vi "GFITS_getKeyvalueFromDatabase.vi"(0 "key name in header":string, 1 "Database RefNum in":T1, 5 "Keyname":string, 7 "comment":string, 9 "extension":i16=1, 11 "error in (no error)":errorcluster) -> (6 "table out":string[][](table), 10 "datatype":u16[](array[numeric]), 14 "function to use":string, 15 "error out":errorcluster)   [LabVIEW 2016]
uses:
  GFITS_datatypesctl.ctl
  DBSHAND/private/vis/DatabaseHand_RefNum.ctl
  DBSHAND/private/vis/DatabaseHand_Element_Get(string).vi
  GFITS_Gbls.vi
  DBSHAND/private/vis/DatabaseHand_Element_Get(3DArr).vi
panel:
  in  "Case Constant\n(See Context Help)":bool
  out "TCSINFO":string[][](array[string])
  in  "ARRINFO":string[][](table)
  out "value":string
  out "response":string
  out "utshut":string
  in  "Types":T2={"TBIT"=1, "TBYTE"=11, "TSTRING"=16, "TSHORT"=21, "TLONG"=41, "TFLOAT"=42, "TDOUBLE"=82, "TCOMPLEX"=83, "TDBLCOMPLEX"=163, "TUINT"=30, "TUSHORT"=20, "TULONG"=40, "TINT"=31, "TSBYTE"=12, "TLONGLONG"=81, "TLOGICAL"=14}
  in  "Supported DataTypes":i32(listbox)
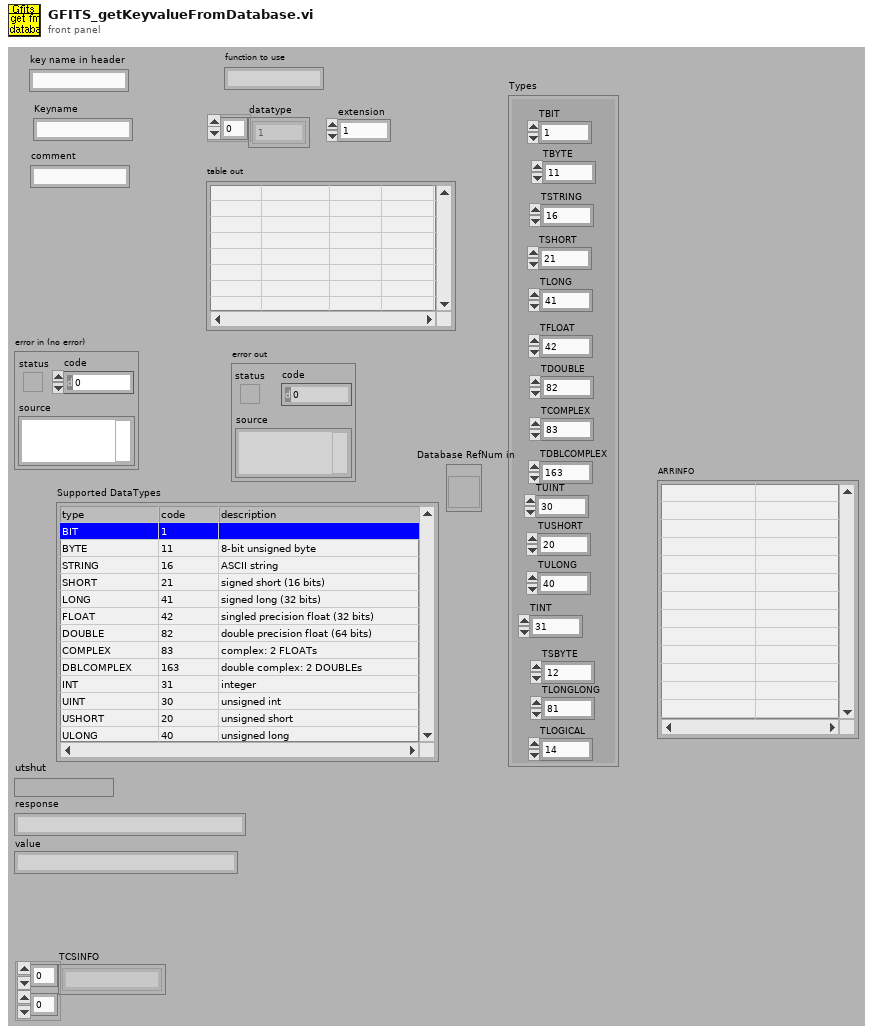
[diagram p1: front panel]
types:
  T1 = typedef "DatabaseHand_RefNum.ctl" = refnum<vi>
  T2 = typedef "GFITS_datatypesctl.ctl" = cluster{"TBIT":i32, "TBYTE":i32, "TSTRING":i32, "TSHORT":i32, "TLONG":i32, "TFLOAT":i32, "TDOUBLE":i32, "TCOMPLEX":i32, "TDBLCOMPLEX":i32, "TUINT":i32, "TUSHORT":i32, "TULONG":i32, "TINT":i32, "TSBYTE":i32, "TLONGLONG":i32, "TLOGICAL":i32}
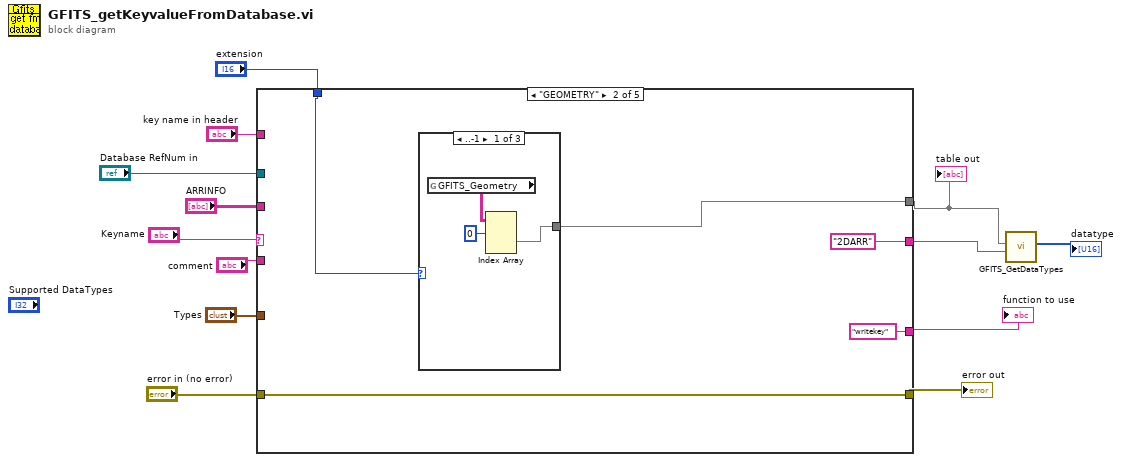
[diagram p0: block diagram]
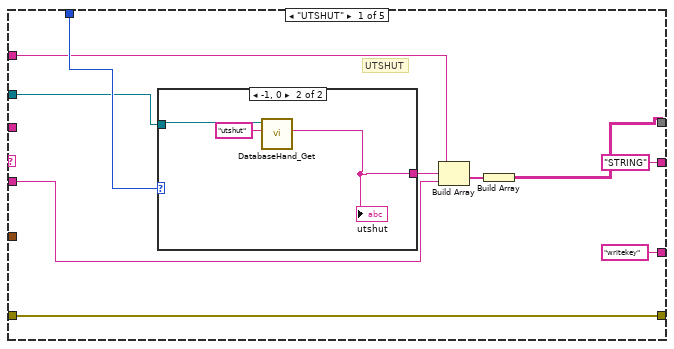
[diagram p2: hidden frame]
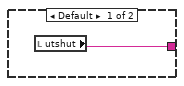
[diagram p3: hidden frame]
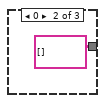
[diagram p4: hidden frame]
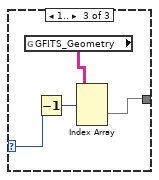
[diagram p5: hidden frame]
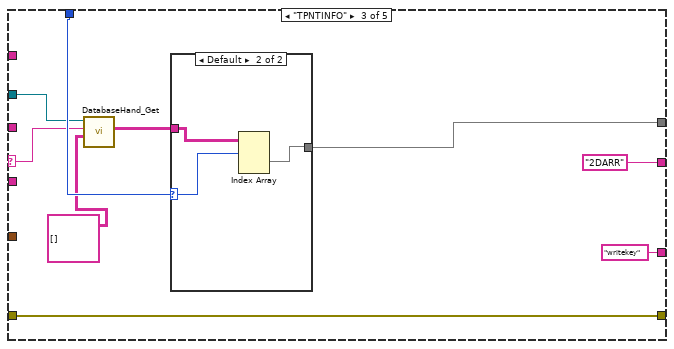
[diagram p6: hidden frame]
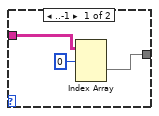
[diagram p7: hidden frame]
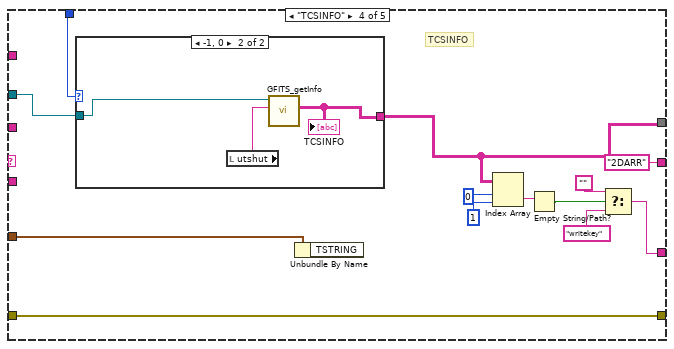
[diagram p8: hidden frame]
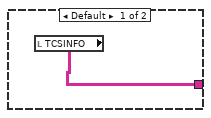
[diagram p9: hidden frame]
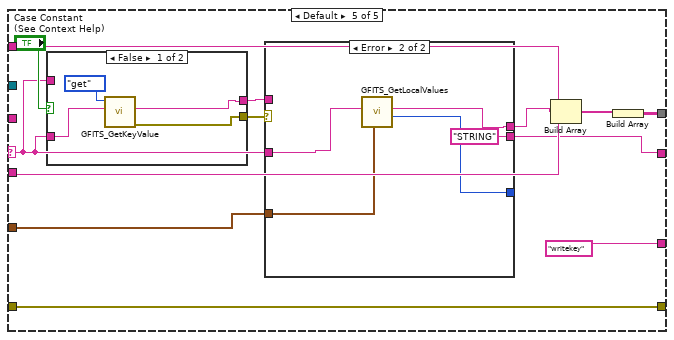
[diagram p10: hidden frame]
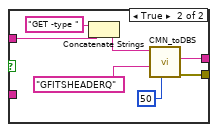
[diagram p11: hidden frame]
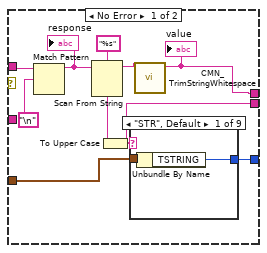
[diagram p12: hidden frame]
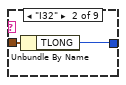
[diagram p13: hidden frame]
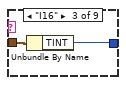
[diagram p14: hidden frame]
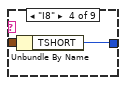
[diagram p15: hidden frame]
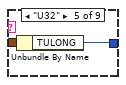
[diagram p16: hidden frame]
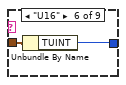
[diagram p17: hidden frame]
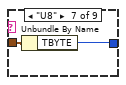
[diagram p18: hidden frame]
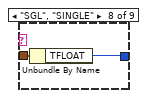
[diagram p19: hidden frame]
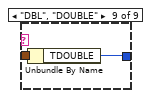
[diagram p20: hidden frame]
diagram:
  n1 = case shown="\"GEOMETRY\"" "Keyname" {
    selector: "Keyname" -> [_ _ w43 _ w74]
    tunnel: "key name in header" -> [w20 _ _ _ w83]
    tunnel: "comment" -> [w19 _ _ _ w82]
    tunnel: "error in (no error)" -> [w17 w32 w49 w68 w85]
    tunnel: [w17 w32 w49 w68 w85] -> w10
    tunnel: ["writekey" "writekey" "writekey" w65 "writekey"] -> w9
    tunnel: [w18 w29 w46 w60 w81] -> w2
    tunnel: "extension" -> [w21 w30 w47 w64 _]
    tunnel: "Types" -> [_ _ _ w58 w78]
    tunnel: "ARRINFO" -> [_ _ _ _ _]
    tunnel: "Database RefNum in" -> [w15 _ w44 w56 _]
    tunnel: ["STRING" ("type") "2DARR" ("type") "2DARR" ("type") "2DARR" ("type") w73] -> w1
    frame "UTSHUT" {
      # "UTSHUT"
      n2 = case shown="-1, 0" w21 {
        tunnel: [w24 w25] -> w22
        tunnel: w15 -> [_ w27]
        frame Default {
          n3 = local read "utshut"() -> (w24:string)
        }
        frame -1, 0 {
          n4 = call-poly "DatabaseHand_Get.vi"("name"="utshut", "Database RefNum in"=w27) -> ("value"=w25:string)  [unwired: 3 in, 6 out]
          "utshut" <- w25
        }
      }
      n5 = Build Array(w20, w22, w19) -> (w23:string[])
      n6 = Build Array(w23) -> (w18:string[][])
    }
    frame "GEOMETRY" {
      n7 = case shown="..-1" w30 {
        selector: w30 -> [_ _ w39]
        tunnel: [w33 string[][] [] ("GFITS_Geometry") w38] -> w29
        frame ..-1 {
          n8 = global read "GFITS_Gbls.vi" "GFITS_Geometry"() -> (w35:string[][][])
          n9 = Index Array(array=w35, index (dim 0)=0 ("index (page)")) -> (element=w33:string[][])  [unwired: 2 in]
        }
        frame 0 {
        }
        frame 1.. {
          n10 = global read "GFITS_Gbls.vi" "GFITS_Geometry"() -> (w40:string[][][])
          n11 = Decrement(x=w39) -> (x-1=w37:i16)
          n12 = Index Array(array=w40, index (dim 0)=w37) -> (element=w38:string[][])  [unwired: 2 in]
        }
      }
    }
    frame "TPNTINFO" {
      n13 = call-poly "DatabaseHand_Get.vi"("default value"=string[][][] [] ("GFITS_Geometry"), "name"=w43, "Database RefNum in"=w44) -> ("value"=w41:string[][][])  [unwired: 2 in, 6 out]
      n14 = case shown="Default" w47 {
        selector: w47 -> [_ w54]
        tunnel: [w51 w55] -> w46
        tunnel: w41 -> [w50 w53]
        frame ..-1 {
          n15 = Index Array(array=w50, index (dim 0)=0 ("index (page)")) -> (element=w51:string[][])  [unwired: 2 in]
        }
        frame Default {
          n16 = Index Array(array=w53, index (dim 0)=w54) -> (element=w55:string[][])  [unwired: 2 in]
        }
      }
    }
    frame "TCSINFO" {
      # "TCSINFO"
      n17 = case shown="-1, 0" w64 {
        tunnel: [w69 w72] -> w60
        tunnel: w56 -> [_ w70]
        frame Default {
          n18 = local read "TCSINFO"() -> (w69:string[][])
        }
        frame -1, 0 {
          n19 = local read "utshut"() -> (w71:string)
          n20 = call "GFITS_getInfo.vi"("ID"=w71, "Database RefNum in"=w70) -> ("INFO"=w72:string[][])  [unwired: 9 out]
          "TCSINFO" <- w72
        }
      }
      n21 = Unbundle By Name(w58) -> ()  [unwired: 1 out]
      n22 = Index Array(array=w60, index (row)=0 ("Index (row)"), index (col)=1 ("disabled index (col)")) -> (element=w61:string)
      n23 = Empty String/Path?(string/path=w61) -> (empty?=w59:bool)
      n24 = Select(t="", s=w59, f="writekey") -> (s? t:f=w65:string)
    }
    frame Default {
      n25 = case shown="False" "Case Constant\n(See Context Help)" {
        tunnel: [w88 w92] -> w80
        tunnel: w74 -> [_ w91]
        tunnel: [w87 w90] -> w77
        tunnel: w74 -> [w89 _]
        frame False {
          n26 = call "GFITS_GetKeyValue.vi"("keyname"=w89, "action"=enum16{"get", "clear"}."get") -> ("error out"=w88:errorcluster, "response"=w87:string)  [unwired: 1 in, 7 out]
        }
        frame True {
          n27 = Concatenate Strings("GET -type ", w91) -> (w93:string)
          n28 = call "CMN_toDBS.vi"("ms timeout (-1)"=50, "response Q"="GFITSHEADERQ", "command"=w93) -> ("error out"=w92:errorcluster, "response"=w90:string)  [unwired: 1 in, 6 out]
        }
      }
      n29 = case shown="Error" w80 {
        tunnel: w77 -> [w102 _]
        tunnel: [w98 w128] -> w79
        tunnel: w78 -> [w105 w126]
        tunnel: [w104 w127] -> _
        tunnel: w74 -> [_ w129]
        tunnel: [w97 "STRING"] -> w73
        frame No Error {
          n30 = Match Pattern(string=w102, regular expression="\n") -> (before substring=w100:string)  [unwired: 4 out]
          "response" <- w100
          n31 = Scan From String(format string="%s", input string=w100) -> (remaining string=w99:string, output 1=w103:string)  [unwired: 2 in, 3 out]
          n32 = To Upper Case(1:w103) -> (0:w97:string)
          n33 = case shown="\"STR\", Default" w97 {
            tunnel: w105 -> [w108 w110 w112 w114 w116 w118 w120 w122 w124]
            tunnel: [w107 w109 w111 w113 w115 w117 w119 w121 w123] -> w104
            frame "STR", Default {
              n34 = Unbundle By Name(w108) -> ("TSTRING"=w107:i32)
            }
            frame "I32" {
              n35 = Unbundle By Name(w110) -> ("TLONG"=w109:i32)
            }
            frame "I16" {
              n36 = Unbundle By Name(w112) -> ("TINT"=w111:i32)
            }
            frame "I8" {
              n37 = Unbundle By Name(w114) -> ("TSHORT"=w113:i32)
            }
            frame "U32" {
              n38 = Unbundle By Name(w116) -> ("TULONG"=w115:i32)
            }
            frame "U16" {
              n39 = Unbundle By Name(w118) -> ("TUINT"=w117:i32)
            }
            frame "U8" {
              n40 = Unbundle By Name(w120) -> ("TBYTE"=w119:i32)
            }
            frame "SGL", "SINGLE" {
              n41 = Unbundle By Name(w122) -> ("TFLOAT"=w121:i32)
            }
            frame "DBL", "DOUBLE" {
              n42 = Unbundle By Name(w124) -> ("TDOUBLE"=w123:i32)
            }
          }
          n43 = call "CMN_TrimStringWhitespace.vi"("string"=w99) -> ("trimmed string"=w98:string)  [unwired: 1 in, 8 out]
          "value" <- w98
        }
        frame Error {
          n44 = call "GFITS_GetLocalValues.vi"("Types"=w126, "key"=w129) -> ("datatype"=w127:u16, "value"=w128:string)  [unwired: 1 in, 7 out]
        }
      }
      n45 = Build Array(w83, w79, w82) -> (w84:string[])
      n46 = Build Array(w84) -> (w81:string[][])
    }
  }
  "error out" <- w10
  "function to use" <- w9
  "table out" <- w2
  n47 = call "GFITS_GetDataTypes.vi"("type"=w1, "keys"=w2) -> ("datatypes"=→"datatype":i32[])  [unwired: 9 out]
